vi "test_F9P_232-2.vi"() -> ()   [LabVIEW 2019] (continued)
08,66,357,,09,08,194,,3*7A\r\n$GBGSV,5,3,17,10,14,222,36,11,34,144,45,13,50,316,22,14,73,036,33,3*77\r\n$GBGSV,5,4,17,16,25,186,36,27,10,317,,28,61,307,,33,75,244,,3*71\r\n$GBGSV,5,5,17,34,11,143,,3*43\r\n$GNGLL,3723.57105,N,12657.01334,E,064952.00,A,A*7A\r\n$GNRMC,064953.00,A,3723.57103,N,12657.01334,E,0.039,,250720,,,A,V*16\r\n$GNVTG,,T,,M,0.039,N,0.072,K,A*32\r\n$GNGGA,064953.00,3723.57103,N,12657.01334,E,1,12,0.62,36.0,M,18.5,M,,*76\r\n$GNGSA,A,3,17,19,06,12,05,02,09,,,,,,1.04,0.62,0.84,1*09\r\n$GNGSA,A,3,85,70,71,72,,,,,,,,,1.04,0.62,0.84,2*06\r\n$GNGSA,A,3,36,19,11,04,09,12,,,,,,,1.04,0.62,0.84,3*0D\r\n$GNGSA,A,3,28,11,14,13,33,08,10,,,,,,1.04,0.62,0.84,4*0D\r\n$GPGSV,4,1,13,02,67,338,26,04,06,036,11,05,50,265,43,06,56,081,45,1*60\r\n$GPGSV,4,2,13,07,08,102,,09,36,055,40,12,17,260,29,13,11,191,30,1*66\r\n$GPGSV,4,3,13,17,16,158,45,19,34,162,41,25,11,291,20,29,09,322,30,1*6F\r\n$GPGSV,4,4,13,30,03,132,,1*56\r\n$GPGSV,4,1,13,02,67,338,,04,06,036,,05,50,265,31,06,56,081,35,6*61\r\n$GPGSV,4,2,13,07,08,102,,09,36,055,26,12,17,260,17,13,11,191,,6*6F\r\n$GPGSV,4,3,13,17,16,158,34,19,34,162,,25,11,291,25,29,09,322,,6*6D\r\n$GPGSV,4,4,13,30,03,132,,6*51\r\n$GLGSV,2,1,06,70,51,030,17,71,72,230,44,72,20,218,36,84,06,136,09,1*77\r\n$GLGSV,2,2,06,85,61,118,45,86,55,338,,1*7B\r\n$GLGSV,2,1,06,70,51,030,,71,72,230,29,72,20,218,34,84,06,136,08,3*7B\r\n$GLGSV,2,2,06,85,61,118,32,86,55,338,,3*79\r\n$GAGSV,3,1,09,02,03,285,11,04,67,079,38,05,00,212,,09,47,197,29,7*7C\r\n$GAGSV,3,2,09,11,78,050,31,12,30,117,35,18,58,277,47,19,15,041,11,7*7E\r\n$GAGSV,3,3,09,36,37,315,22,7*4C\r\n$GAGSV,3,1,09,02,03,285,,04,67,079,29,05,00,212,,09,47,197,41,2*77\r\n$GAGSV,3,2,09,11,78,050,30,12,30,117,32,18,58,277,34,19,15,041,,2*79\r\n$GAGSV,3,3,09,36,37,315,29,2*42\r\n$GBGSV,5,1,17,01,42,153,,03,45,207,,04,35,133,,05,09,257,,1*7C\r\n$GBGSV,5,2,17,06,29,183,,07,08,201,,08,66,357,25,09,08,194,,1*7F\r\n$GBGSV,5,3,17,10,14,222,36,11,34,144,33,13,50,316,32,14,73,036,31,1*77\r\n$GBGSV,5,4,17,16,25,186,,27,10,317,,28,61,307,34,33,75,247,43,1*75\r\n$GBGSV,5,5,17,34,11,143,11,1*41\r\n$GBGSV,5,1,17,01,42,153,,03,45,207,,04,35,133,,05,09,257,,3*7E\r\n$GBGSV,5,2,17,06,29,183,,07,08,201,,08,66,357,,09,08,194,,3*7A\r\n$GBGSV,5,3,17,10,14,222,38,11,34,144,45,13,50,316,22,14,73,036,32,3*78\r\n$GBGSV,5,4,17,16,25,186,35,27,10,317,,28,61,307,,33,75,247,,3*71\r\n$GBGSV,5,5,17,34,11,143,,3*43\r\n$GNGLL,3723.57103,N,12657.01334,E,064953.00,A,A*7D\r\n$GNRMC,064954.00,A,3723.57095,N,12657.01327,E,0.435,279.25,250720,,,A,V*00\r\n$GNVTG,279.25,T,,M,0.435,N,0.807,K,A*25\r\n$GNGGA,064954.00,3723.57095,N,12657.01327,E,1,12,0.65,36.0,M,18.5,M,,*7A\r\n$GNGSA,A,3,17,19,06,12,05,02,09,,,,,,1.11,0.65,0.90,1*0F\r\n$GNGSA,A,3,85,70,71,72,,,,,,,,,1.11,0.65,0.90,2*00\r\n$GNGSA,A,3,36,19,11,04,09,12,,,,,,,1.11,0.65,0.90,3*0B\r\n$GNGSA,A,3,28,11,14,13,33,08,10,,,,,,1.11,0.65,0.90,4*0B\r\n$GPGSV,4,1,13,02,67,338,26,04,06,036,14,05,50,265,45,06,56,081,44,1*62\r\n$GPGSV,4,2,13,07,08,102,,09,36,055,38,12,17,260,27,13,11,191,32,1*65\r\n$GPGSV,4,3,13,17,16,158,43,19,34,162,34,25,11,291,30,29,09,322,29,1*62\r\n$GPGSV,4,4,13,30,03,132,,1*56\r\n$GPGSV,4,1,13,02,67,338,,04,06,036,19,05,50,265,31,06,56,081,34,6*68\r\n$GPGSV,4,2,13,07,08,102,,09,36,055,32,12,17,260,18,13,11,191,,6*65\r\n$GPGSV,4,3,13,17,16,158,24,19,34,162,,25,11,291,24,29,09,322,22,6*6D\r\n$GPGSV,4,4,13,30,03,132,,6*51\r\n$GLGSV,2,1,06,70,51,030,19,71,72,230,40,72,20,218,44,84,06,136,07,1*76\r\n$GLGSV,2,2,06,85,61,118,38,86,55,338,,1*71\r\n$GLGSV,2,1,06,70,51,030,,71,72,230,29,72,20,218,36,84,06,136,12,3*72\r\n$GLGSV,2,2,06,85,61,118,32,86,55,338,,3*79\r\n$GAGSV,3,1,09,02,03,285,11,04,67,079,42,05,00,212,,09,47,197,40,7*7E\r\n$GAGSV,3,2,09,11,78,050,33,12,30,117,31,18,58,277,46,19,15,041,12,7*7A\r\n$GAGSV,3,3,09,36,37,315,23,7*4D\r\n$GAGSV,3,1,09,02,03,285,,04,67,079,34,05,00,212,,09,47,197,40,2*7A\r\n$GAGSV,3,2,09,11,78,050,32,12,30,117,35,18,58,277,37,19,15,041,,2*7F\r\n$GAGSV,3,3,09,36,37,315,30,2*4A\r\n$GBGSV,5,1,17,01,42,153,,03,45,207,,04,35,133,,05,09,257,,1*7C\r\n$GBGSV,5,2,17,06,29,183,,07,08,201,,08,66,357,25,09,08,194,,1*7F\r\n$GBGSV,5,3,17,10,14,222,44,11,34,144,42,13,50,316,32,14,73,036,38,1*7D\r\n$GBGSV,5,4,17,16,25,186,27,27,10,317,,28,61,307,37,33,75,247,44,1*74\r\n$GBGSV,5,5,17,34,10,143,,1*40\r\n$GBGSV,5,1,17,01,42,153,,03,45,207,,04,35,133,,05,09,257,,3*7E\r\n$GBGSV,5,2,17,06,29,183,,07,08,201,,08,66,357,,09,08,194,,3*7A\r\n$GBGSV,5,3,17,10,14,222,40,11,34,144,43,13,50,316,22,14,73,036,38,3*7B\r\n$GBGSV,5,4,17,16,25,186,27,27,10,317,,28,61,307,,33,75,247,,3*72\r\n$GBGSV,5,5,17,34,10,143,,3*42\r\n$GNGLL,3723.57095,N,12657.01327,E,064954.00,A,A*76\r\n$GNRMC,064955.00,A,3723.57087,N,12657.01326,E,0.059,,250720,,,A,V*18\r\n$GNVTG,,T,,M,0.059,N,0.109,K,A*39\r\n$GNGGA,064955.00,3723.57087,N,12657.01326,E,1,12,0.74,36.2,M,18.5,M,,*7B\r\n$GNGSA,A,3,17,19,06,12,05,02,09,,,,,,1.34,0.74,1.12,1*03\r\n$GNGSA,A,3,85,71,72,,,,,,,,,,1.34,0.74,1.12,2*0B\r\n$GNGSA,A,3,36,11,04,09,12,,,,,,,,1.34,0.74,1.12,3*0F\r\n$GNGSA,A,3,28,11,14,13,33,08,10,,,,,,1.34,0.74,1.12,4*07\r\n$GPGSV,4,1,13,02,67,338,33,04,06,036,14,05,50,265,45,06,56,081,44,1*66\r\n$GPGSV,4,2,13,07,08,102,22,09,36,055,40,12,17,260,31,13,11,191,30,1*6F\r\n$GPGSV,4,3,13,17,16,158,45,19,34,162,39,25,11,291,30,29,09,322,34,1*65\r\n$GPGSV,4,4,13,30,03,132,,1*56\r\n$GPGSV,4,1,13,02,67,338,,04,06,036,18,05,50,265,35,06,56,081,36,6*6F\r\n$GPGSV,4,2,13,07,08,102,,09,36,055,39,12,17,260,22,13,11,191,,6*67\r\n$GPGSV,4,3,13,17,16,158,25,19,34,162,,25,11,291,21,29,09,322,26,6*6D\r\n$GPGSV,4,4,13,30,03,132,,6*51\r\n$GLGSV,2,1,06,70,51,030,,71,72,230,40,72,20,218,37,84,06,136,11,1*7D\r\n$GLGSV,2,2,06,85,61,118,35,86,55,338,,1*7C\r\n$GLGSV,2,1,06,70,51,030,,71,72,230,20,72,20,218,35,84,06,136,08,3*73\r\n$GLGSV,2,2,06,85,61,118,31,86,55,338,,3*7A\r\n$GAGSV,3,1,09,02,03,285,08,04,67,079,42,05,00,212,,09,47,197,36,7*77\r\n$GAGSV,3,2,09,11,78,050,32,12,30,117,31,18,58,277,49,19,15,041,09,7*7E\r\n$GAGSV,3,3,09,36,37,315,30,7*4F\r\n$GAGSV,3,1,09,02,03,285,,04,67,079,37,05,00,212,,09,47,197,40,2*79\r\n$GAGSV,3,2,09,11,78,050,33,12,30,117,36,18,58,277,41,19,15,041,,2*7C\r\n$GAGSV,3,3,09,36,37,315,21,2*4A\r\n$GBGSV,5,1,17,01,42,153,,03,45,207,,04,35,133,,05,09,257,,1*7C\r\n$GBGSV,5,2,17,06,29,183,,07,08,201,,08,66,357,26,09,08,194,,1*7C\r\n$GBGSV,5,3,17,10,14,222,42,11,34,144,36,13,50,316,31,14,73,036,35,1*76\r\n$GBGSV,5,4,17,16,25,186,31,27,10,317,,28,61,307,39,33,75,247,44,1*7D\r\n$GBGSV,5,5,17,34,10,143,,1*40\r\n$GBGSV,5,1,17,01,42,153,,03,45,207,,04,35,133,,05,09,257,,3*7E\r\n$GBGSV,5,2,17,06,29,183,,07,08,201,,08,66,357,31,09,08,194,,3*78\r\n$GBGSV,5,3,17,10,14,222,41,11,34,144,44,13,50,316,23,14,73,036,39,3*7D\r\n$GBGSV,5,4,17,16,25,186,33,27,10,317,,28,61,307,,33,75,247,,3*77\r\n$GBGSV,5,5,17,34,10,143,,3*42\r\n$GNGLL,3723.57087,N,12657.01326,E,064955.00,A,A*75\r\n$GNRMC,064956.00,A,3723.57085,N,12657.01331,E,0.135,,250720,,,A,V*14\r\n$GNVTG,,T,,M,0.135,N,0.250,K,A*3D\r\n$GNGGA,064956.00,3723.57085,N,12657.01331,E,1,12,0.71,36.2,M,18.5,M,,*79\r\n$GNGSA,A,3,17,19,06,12,05,02,09,,,,,,1.26,0.71,1.04,1*02\r\n$GNGSA,A,3,85,71,72,,,,,,,,,,1.26,0.71,1.04,2*0A\r\n$GNGSA,A,3,36,11,04,09,12,,,,,,,,1.26,0.71,1.04,3*0E\r\n$GNGSA,A,3,28,11,14,13,33,08,10,,,,,,1.26,0.71,1.04,4*06\r\n$GPGSV,4,1,13,02,67,338,33,04,06,036,14,05,50,265,42,06,56,081,43,1*66\r\n$GPGSV,4,2,13,07,08,102,,09,36,055,41,12,17,260,30,13,11,191,28,1*66\r\n$GPGSV,4,3,13,17,16,158,45,19,34,162,39,25,11,291,31,29,09,322,35,1*65\r\n$GPGSV,4,4,13,30,03,132,,1*56\r\n$GPGSV,4,1,13,02,67,338,,04,06,036,17,05,50,265,35,06,56,081,38,6*6E\r\n$GPGSV,4,2,13,07,08,102,,09,36,055,38,12,17,260,23,13,11,191,,6*67\r\n$GPGSV,4,3,13,17,16,158,23,19,34,162,,25,11,291,18,29,09,322,26,6*61\r\n$GPGSV,4,4,13,30,03,132,,6*51\r\n$GLGSV,2,1,06,70,51,030,25,71,72,230,40,72,20,218,39,84,06,136,08,1*7C\r\n$GLGSV,2,2,06,85,61,118,38,86,55,338,,1*71\r\n$GLGSV,2,1,06,70,51,030,,71,72,230,29,72,20,218,33,84,06,136,09,3*7D\r\n$GLGSV,2,2,06,85,61,118,29,86,55,338,,3*73\r\n$GAGSV,3,1,09,02,03,285,11,04,67,079,41,05,00,212,,09,47,197,29,7*72\r\n$GAGSV,3,2,09,11,78,050,32,12,30,117,31,18,58,277,48,19,15,041,09,7*7F\r\n$GAGSV,3,3,09,36,37,315,30,7*4F\r\n$GAGSV,3,1,09,02,03,285,,04,67,079,37,05,00,212,,09,47,197,39,2*77\r\n$GAGSV,3,2,09,11,78,050,32,12,30,117,36,18,58,277,44,19,15,041,,2*78\r\n$GAGSV,3,3,09,36,37,315,21,2*4A\r\n$GBGSV,5,1,17,01,42,153,,03,45,207,,04,35,133,,05,09,257,,1*7C\r\n$GBGSV,5,2,17,06,29,183,,07,08,201,,08,66,357,27,09,08,194,,1*7D\r\n$GBGSV,5,3,17,10,14,222,43,11,34,144,37,13,50,316,32,14,73,036,36,1*76\r\n$GBGSV,5,4,17,16,25,186,35,27,10,317,,28,61,307,39,33,75,247,45,1*78\r\n$GBGSV,5,5,17,34,10,143,,1*40\r\n$GBGSV,5,1,17,01,42,153,,03,45,207,,04,35,133,,05,09,257,,3*7E\r\n$GBGSV,5,2,17,06,29,183,,07,08,201,,08,66,357,33,09,08,194,,3*7A\r\n$GBGSV,5,3,17,10,14,222,36,11,34,144,43,13,50,316,22,14,73,036,39,3*7B\r\n$GBGSV,5,4,17,16,25,186,33,27,10,317,,28,61,307,,33,75,247,,3*77\r\n$GBGSV,5,5,17,34,10,143,,3*42\r\n$GNGLL,3723.57085,N,12657.01331,E,064956.00,A,A*72\r\n$GNRMC,064957.00,A,3723.57091,N,12657.01330,E,0.381,,250720,,,A,V*1C\r\n$GNVTG,,T,,M,0.381,N,0.706,K,A*36\r\n$GNGGA,064957.00,3723.57091,N,12657.01330,E,1,12,0.71,36.3,M,18.5,M,,*7D\r\n$GNGSA,A,3,17,19,06,12,05,02,09,,,,,,1.26,0.71,1.04,1*02\r\n$GNGSA,A,3,85,71,72,,,,,,,,,,1.26,0.71,1.04,2*0A\r\n$GNGSA,A,3,36,11,04,09,12,,,,,,,,1.26,0.71,1.04,3*0E\r\n$GNGSA,A,3,28,11,14,13,33,08,10,,,,,,1.26,0.71,1.04,4*06\r\n$GPGSV,4,1,13,02,67,338,33,04,06,036,14,05,50,265,44,06,56,081,27,1*62\r\n$GPGSV,4,2,13,07,08,102,,09,36,055,32,12,17,260,24,13,11,191,28,1*67\r\n$GPGSV,4,3,13,17,16,158,46,19,34,162,36,25,11,291,27,29,09,322,28,1*62\r\n$GPGSV,4,4,13,30,03,132,,1*56\r\n$GPGSV,4,1,13,02,67,338,,04,06,036,15,05,50,265,34,06,56,081,29,6*6D\r\n$GPGSV,4,2,13,07,08,102,,09,36,055,33,12,17,260,22,13,11,191,,6*6D\r\n$GPGSV,4,3,13,17,16,158,36,19,34,162,,25,11,291,17,29,09,322,30,6*6D\r\n$GPGSV,4,4,13,30,03,132,,6*51\r\n$GLGSV,2,1,06,70,51,030,,71,72,230,38,72,20,218,35,84,06,136,07,1*77\r\n$GLGSV,2,2,06,85,61,118,36,86,55,338,,1*7F\r\n$GLGSV,2,1,06,70,51,030,,71,72,230,29,72,20,218,32,84,06,136,07,3*72\r\n$GLGSV,2,2,06,85,61,118,33,86,55,338,,3*78\r\n$GAGSV,3,1,09,02,03,285,07,04,67,079,26,05,00,212,,09,47,197,39,7*75\r\n$GAGSV,3,2,09,11,78,050,34,12,30,117,25,18,58,277,42,19,15,041,08,7*77\r\n$GAGSV,3,3,09,36,37,315,34,7*4B\r\n$GAGSV,3,1,09,02,03,285,,04,67,079,34,05,00,212,,09,47,197,35,2*78\r\n$GAGSV,3,2,09,11,78,050,23,12,30,117,21,18,58,277,39,19,15,041,,2*74\r\n$GAGSV,3,3,09,36,37,315,32,2*48\r\n$GBGSV,5,1,17,01,42,153,,03,45,207,,04,35,133,,05,09,257,,1*7C\r\n$GBGSV,5,2,17,06,29,183,,07,08,201,,08,66,357,28,09,08,194,,1*72\r\n$GBGSV,5,3,17,10,14,222,37,11,34,144,30,13,50,316,34,14,73,036,34,1*76\r\n$GBGSV,5,4,17,16,25,186,32,27,10,317,,28,61,307,41,33,75,247,43,1*76\r\n$GBGSV,5,5,17,34,10,143,,1*40\r\n$GBGSV,5,1,17,01,42,153,,03,45,207,,04,35,133,,05,09,257,,3*7E\r\n$GBGSV,5,2,17,06,29,183,,07,08,201,,08,66,357,26,09,08,194,,3*7E\r\n$GBGSV,5,3,17,10,14,222,31,11,34,144,39,13,50,316,30,14,73,036,29,3*73\r\n$GBGSV,5,4,17,16,25,186,36,27,10,317,,28,61,307,,33,75,247,,3*72\r\n$GBGSV,5,5,17,34,10,143,,3*42\r\n$GNGLL,3723.57091,N,12657.01330,E,064957.00,A,A*77\r\n$GNRMC,064958.00,A,3723.57093,N,12657.01327,E,0.089,,250720,,,A,V*1C\r\n$GNVTG,,T,,M,0.089,N,0.165,K,A*3E\r\n$GNGGA,064958.00,3723.57093,N,12657.01327,E,1,12,0.62,36.4,M,18.5,M,,*73\r\n$GNGSA,A,3,17,19,06,12,05,02,09,,,,,,1.04,0.62,0.84,1*09\r\n$GNGSA,A,3,85,71,72,,,,,,,,,,1.04,0.62,0.84,2*01\r\n$GNGSA,A,3,36,19,11,04,09,12,,,,,,,1.04,0.62,0.84,3*0D\r\n$GNGSA,A,3,28,11,14,13,33,08,10,,,,,,1.04,0.62,0.84,4*0D\r\n$GPGSV,4,1,13,02,67,338,34,04,06,036,14,05,50,265,32,06,56,081,26,1*65\r\n$GPGSV,4,2,13,07,08,102,,09,36,055,26,12,17,260,24,13,11,191,27,1*6D\r\n$GPGSV,4,3,13,17,16,158,41,19,34,162,25,25,11,291,30,29,09,322,28,1*61\r\n$GPGSV,4,4,13,30,03,132,,1*56\r\n$GPGSV,4,1,13,02,67,338,,04,06,036,,05,50,265,30,06,56,081,33,6*66\r\n$GPGSV,4,2,13,07,08,102,,09,36,055,35,12,17,260,23,13,11,191,,6*6A\r\n$GPGSV,4,3,13,17,16,158,36,19,34,162,,25,11,291,17,29,09,322,30,6*6D\r\n$GPGSV,4,4,13,30,03,132,,6*51\r\n$GLGSV,2,1,06,70,51,030,,71,72,230,33,72,20,218,39,84,06,136,08,1*7F\r\n$GLGSV,2,2,06,85,61,118,33,86,55,338,,1*7A\r\n$GLGSV,2,1,06,70,51,030,,71,72,230,22,72,20,218,31,84,06,136,10,3*7C\r\n$GLGSV,2,2,06,85,61,118,33,86,55,338,,3*78\r\n$GAGSV,3,1,09,02,03,285,12,04,67,079,28,05,00,212,,09,47,197,32,7*74\r\n$GAGSV,3,2,09,11,78,050,22,12,30,117,23,18,58,277,35,19,15,041,09,7*77\r\n$GAGSV,3,3,09,36,37,315,23,7*4D\r\n$GAGSV,3,1,09,02,03,285,,04,67,079,29,05,00,212,,09,47,197,38,2*79\r\n$GAGSV,3,2,09,11,78,050,23,12,30,117,24,18,58,277,37,19,15,041,,2*7F\r\n$GAGSV,3,3,09,36,37,315,35,2*4F\r\n$GBGSV,5,1,17,01,42,153,,03,45,207,,04,35,133,,05,09,257,,1*7C\r\n$GBGSV,5,2,17,06,29,183,,07,08,201,,08,66,357,26,09,08,194,,1*7C\r\n$GBGSV,5,3,17,10,14,222,33,11,34,144,20,13,50,316,30,14,73,036,23,1*71\r\n$GBGSV,5,4,17,16,25,186,31,27,10,317,,28,61,307,35,33,75,247,36,1*74\r\n$GBGSV,5,5,17,34,10,143,,1*40\r\n$GBGSV,5,1,17,01,42,153,,03,45,207,,04,35,133,,05,09,257,,3*7E\r\n$GBGSV,5,2,17,06,29,183,,07,08,201,,08,66,357,28,09,08,194,,3*70\r\n$GBGSV,5,3,17,10,14,222,31,11,34,144,43,13,50,316,30,14,73,036,28,3*7F\r\n$GBGSV,5,4,17,16,25,186,32,27,10,317,,28,61,307,,33,75,247,,3*76\r\n$GBGSV,5,5,17,34,10,143,,3*42\r\n$GNGLL,3723.57093,N,12657.01327,E,064958.00,A,A*7C\r\n$GNRMC,064959.00,A,3723.57094,N,12657.01328,E,0.093,,250720,,,A,V*1E\r\n$GNVTG,,T,,M,0.093,N,0.172,K,A*33\r\n$GNGGA,064959.00,3723.57094,N,12657.01328,E,1,12,0.74,36.3,M,18.5,M,,*7A\r\n$GNGSA,A,3,17,19,06,12,05,02,09,,,,,,1.34,0.74,1.12,1*03\r\n$GNGSA,A,3,85,71,72,,,,,,,,,,1.34,0.74,1.12,2*0B\r\n$GNGSA,A,3,36,11,04,09,12,,,,,,,,1.34,0.74,1.12,3*0F\r\n$GNGSA,A,3,28,11,14,13,33,08,10,,,,,,1.34,0.74,1.12,4*07\r\n$GPGSV,4,1,13,02,67,338,34,04,06,036,13,05,50,265,35,06,56,081,31,1*63\r\n$GPGSV,4,2,13,07,08,102,,09,36,055,28,12,17,260,24,13,11,191,24,1*60\r\n$GPGSV,4,3,13,17,16,158,38,19,34,162,34,25,11,291,22,29,09,322,24,1*60\r\n$GPGSV,4,4,13,30,03,132,,1*56\r\n$GPGSV,4,1,13,02,67,338,,04,06,036,,05,50,265,38,06,56,081,35,6*68\r\n$GPGSV,4,2,13,07,08,102,,09,36,055,36,12,17,260,22,13,11,191,,6*68\r\n$GPGSV,4,3,13,17,16,158,35,19,34,162,,25,11,291,18,29,09,322,29,6*69\r\n$GPGSV,4,4,13,30,03,132,,6*51\r\n$GLGSV,2,1,06,70,51,030,,71,72,230,31,72,20,218,23,84,06,136,06,1*78\r\n$GLGSV,2,2,06,85,61,118,35,86,55,338,,1*7C\r\n$GLGSV,2,1,06,70,51,030,,71,72,230,33,72,20,218,26,84,06,136,10,3*7A\r\n$GLGSV,2,2,06,85,61,118,29,86,55,338,,3*73\r\n$GAGSV,3,1,09,02,03,285,10,04,67,079,34,05,00,212,,09,47,197,38,7*71\r\n$GAGSV,3,2,09,11,78,050,22,12,30,117,25,18,58,277,36,19,15,041,,7*7B\r\n$GAGSV,3,3,09,36,37,315,26,7*48\r\n$GAGSV,3,1,09,02,03,285,,04,67,079,29,05,00,212,,09,47,197,37,2*76\r\n$GAGSV,3,2,09,11,78,050,23,12,30,117,32,18,58,277,38,19,15,041,,2*77\r\n$GAGSV,3,3,09,36,37,315,32,2*48\r\n$GBGSV,5,1,17,01,42,153,,03,45,207,,04,35,133,,05,09,257,,1*7C\r\n$GBGSV,5,2,17,06,29,183,,07,08,201,,08,66,357,26,09,08,194,,1*7C\r\n$GBGSV,5,3,17,10,14,222,33,11,34,144,23,13,50,316,23,14,73,036,23,1*70\r\n$GBGSV,5,4,17,16,25,186,28,27,10,317,,28,61,307,31,33,75,247,33,1*7D\r\n$GBGSV,5,5,17,34,10,143,,1*40\r\n$GBGSV,5,1,17,01,42,153,,03,45,207,,04,35,133,,05,09,257,,3*7E\r\n$GBGSV,5,2,17,06,29,183,,07,08,201,,08,66,357,30,09,08,194,,3*79\r\n$GBGSV,5,3,17,10,14,222,35,11,34,144,39,13,50,316,25,14,73,036,18,3*71\r\n$GBGSV,5,4,17,16,25,186,33,27,10,317,,28,61,307,,33,75,247,,3*77\r\n$GBGSV,5,5,17,34,10,143,,3*42\r\n$GNGLL,3723.57094,N,12657.01328,E,064959.00,A,A*75\r\n$GNRMC,065000.00,A,3723.57092,N,12657.01329,E,0.102,,250720,,,A,V*14\r\n$GNVTG,,T,,M,0.102,N,0.189,K,A*3E\r\n$GNGGA,065000.00,3723.57092,N,12657.01329,E,1,12,0.74,36.4,M,18.5,M,,*7E\r\n$GNGSA,A,3,17,19,06,12,05,02,09,,,,,,1.34,0.74,1.12,1*03\r\n$GNGSA,A,3,85,71,72,,,,,,,,,,1.34,0.74,1.12,2*0B\r\n$GNGSA,A,3,36,11,04,09,12,,,,,,,,1.34,0.74,1.12,3*0F\r\n$GNGSA,A,3,28,11,14,13,33,08,10,,,,,,1.34,0.74,1.12,4*07\r\n$GPGSV,4,1,13,02,67,338,33,04,06,036,10,05,50,265,35,06,56,081,27,1*60\r\n$GPGSV,4,2,13,07,08,102,,09,36,055,30,12,17,260,21,13,11,191,26,1*6E\r\n$GPGSV,4,3,13,17,16,158,36,19,34,162,32,25,11,291,25,29,09,322,31,1*6B\r\n$GPGSV,4,4,13,30,03,132,,1*56\r\n$GPGSV,4,1,13,02,67,338,,04,06,036,,05,50,265,35,06,56,081,35,6*65\r\n$GPGSV,4,2,13,07,08,102,,09,36,055,35,12,17,260,20,13,11,191,,6*69\r\n$GPGSV,4,3,13,17,16,158,33,19,34,162,,25,11,291,19,29,09,322,27,6*60\r\n$GPGSV,4,4,13,30,03,132,,6*51\r\n$GLGSV,2,1,06,70,51,030,,71,72,230,33,72,20,218,35,84,06,136,07,1*7C\r\n$GLGSV,2,2,06,85,61,118,37,86,55,338,,1*7E\r\n$GLGSV,2,1,06,70,51,030,,71,72,230,29,72,20,218,31,84,06,136,09,3*7F\r\n$GLGSV,2,2,06,85,61,118,28,86,55,338,,3*72\r\n$GAGSV,3,1,09,02,03,285,09,04,67,079,35,05,00,212,,09,47,197,40,7*77\r\n$GAGSV,3,2,09,11,78,050,31,12,30,117,25,18,58,277,40,19,15,041,,7*78\r\n$GAGSV,3,3,09,36,37,315,26,7*48\r\n$GAGSV,3,1,09,02,03,285,,04,67,079,34,05,00,212,,09,47,197,36,2*7B\r\n$GAGSV,3,2,09,11,78,050,20,12,30,117,33,18,58,277,40,19,15,041,,2*7A\r\n$GAGSV,3,3,09,36,37,315,31,2*4B\r\n$GBGSV,5,1,17,01,42,153,,03,45,207,,04,35,133,,05,09,257,,1*7C\r\n$GBGSV,5,2,17,06,29,183,,07,08,201,,08,66,357,23,09,08,194,,1*79\r\n$GBGSV,5,3,17,10,14,222,28,11,34,144,30,13,50,316,31,14,73,036,31,1*78\r\n$GBGSV,5,4,17,16,25,186,34,27,10,317,,28,61,307,33,33,75,247,34,1*75\r\n$GBGSV,5,5,17,34,10,143,,1*40\r\n$GBGSV,5,1,17,01,42,153,,03,45,207,,04,35,133,,05,09,257,,3*7E\r\n$GBGSV,5,2,17,06,29,183,,07,08,201,,08,66,357,29,09,08,194,,3*71\r\n$GBGSV,5,3,17,10,14,222,36,11,34,144,41,13,50,316,25,14,73,036,20,3*76\r\n$GBGSV,5,4,17,16,25,186,33,27,10,317,,28,61,307,,33,75,247,,3*77\r\n$GBGSV,5,5,17,34,10,143,,3*42\r\n$GNGLL,3723.57092,N,12657.01329,E,065000.00,A,A*76\r\n$GNRMC,065001.00,A,3723.57091,N,12657.01328,E,0.070,,250720,,,A,V*13\r\n$GNVTG,,T,,M,0.070,N,0.129,K,A*30\r\n$GNGGA,065001.00,3723.57091,N,12657.01328,E,1,12,0.85,36.4,M,18.5,M,,*73\r\n$GNGSA,A,3,17,19,06,12,05,02,09,,,,,,1.53,0.85,1.27,1*0A\r\n$GNGSA,A,3,85,71,72,,,,,,,,,,1.53,0.85,1.27,2*02\r\n$GNGSA,A,3,36,11,04,09,12,,,,,,,,1.53,0.85,1.27,3*06\r\n$GNGSA,A,3,28,11,14,13,33,08,10,,,,,,1.53,0.85,1.27,4*0E\r\n$GPGSV,4,1,13,02,67,338,35,04,06,036,09,05,50,265,39,06,56,081,36,1*62\r\n$GPGSV,4,2,13,07,08,102,,09,36,055,33,12,17,260,27,13,11,191,28,1*65\r\n$GPGSV,4,3,13,17,16,158,39,19,34,162,33,25,11,291,26,29,09,322,26,1*60\r\n$GPGSV,4,4,13,30,03,132,,1*56\r\n$GPGSV,4,1,13,02,67,338,,04,06,036,,05,50,265,32,06,56,081,30,6*67\r\n$GPGSV,4,2,13,07,08,102,,09,36,055,39,12,17,260,21,13,11,191,,6*64\r\n$GPGSV,4,3,13,17,16,158,35,19,34,162,,25,11,291,20,29,09,322,27,6*6C\r\n$GPGSV,4,4,13,30,03,132,,6*51\r\n$GLGSV,2,1,06,70,51,030,,71,72,230,38,72,20,218,36,84,06,136,08,1*7B\r\n$GLGSV,2,2,06,85,61,118,38,86,55,338,,1*71\r\n$GLGSV,2,1,06,70,51,030,,71,72,230,29,72,20,218,33,84,06,136,10,3*75\r\n$GLGSV,2,2,06,85,61,118,26,86,55,338,,3*7C\r\n$GAGSV,3,1,09,02,03,285,07,04,67,079,35,05,00,212,,09,47,197,37,7*79\r\n$GAGSV,3,2,09,11,78,050,30,12,30,117,27,18,58,277,36,19,15,041,,7*7A\r\n$GAGSV,3,3,09,36,37,315,25,7*4B\r\n$GAGSV,3,1,09,02,03,285,,04,67,079,31,05,00,212,,09,47,197,35,2*7D\r\n$GAGSV,3,2,09,11,78,050,29,12,30,117,31,18,58,277,27,19,15,041,,2*70\r\n$GAGSV,3,3,09,36,37,315,30,2*4A\r\n$GBGSV,5,1,17,01,42,153,,03,45,207,,04,35,133,,05,09,257,,1*7C\r\n$GBGSV,5,2,17,06,29,183,,07,08,201,,08,66,357,22,09,08,194,,1*78\r\n$GBGSV,5,3,17,10,14,222,27,11,34,144,31,13,50,316,25,14,73,036,34,1*76\r\n$GBGSV,5,4,17,16,25,186,35,27,10,317,,28,61,307,28,33,75,247,37,1*7D\r\n$GBGSV,5,5,17,34,10,143,,1*40\r\n$GBGSV,5,1,17,01,42,153,,03,45,207,,04,35,133,,05,09,257,,3*7E\r\n$GBGSV,5,2,17,06,29,183,,07,08,201,,08,66,357,21,09,08,194,,3*79\r\n$GBGSV,5,3,17,10,14,222,41,11,34,144,39,13,50,316,24,14,73,036,29,3*71\r\n$GBGSV,5,4,17,16,25,186,33,27,10,317,,28,61,307,,33,75,247,,3*77\r\n$GBGSV,5,5,17,34,10,143,,3*42\r\n$GNGLL,3723.57091,N,12657.01328,E,065001.00,A,A*75\r\n$GNRMC,065002.00,A,3723.57089,N,12657.01324,E,0.119,,250720,,,A,V*1B\r\n$GNVTG,,T,,M,0.119,
